vi "状态告警区.vi"(11 "数组":u16[](array[numeric]) format="%04xH") -> (2 "状态告警区 2":T1 {"工作状态" items=["空闲"=0, "水样测试"=1, "标样核查"=2, "零点核查"=3, "跨度核查"=4, "空白测试"=5, "平行样测试"=6, "加标回收"=7, "空白校准"=8, "标样校准"=9, "初始化（清洗）"=10, "单步调试"=254, "简易步骤"=255]; "告警代码" items=["无告警", "缺试剂告警", "缺水样告警", "缺蒸馏水告警", "缺标液告警", "仪表漏液告警", "标定异常告警", "超量程告警", "加热异常", "低试剂预警", "超上限告警", "超下限告警", "仪表内部其他异常", "滴定异常告警", "电极异常告警", "量程切换告警", "参数设置告警", "PH电极电位异常", "电导率电极异常", "浊度光度异常", "溶解氧电极异常", "溶解氧光强异常", "温度异常告警", "PH异常告警", "溶解氧异常告警", "电导率异常告警", "浊度异常告警", "叶绿素异常告警", "藻密度异常告警", "蓝绿藻异常告警", "ORP异常告警", "氨氮异常告警", "清洁刷异常告警", "SD卡异常告警", "蓝牙异常告警", "Wifi异常告警", "流程异常告警"]; "故障代码" items=["无故障", "电机故障", "温度故障", "通讯故障", "滴定故障"]}, 3 "状态告警区":T2 {"工作状态" items=["空闲"=0, "水样测试"=1, "标样核查"=2, "零点核查"=3, "跨度核查"=4, "空白测试"=5, "平行样测试"=6, "加标回收"=7, "空白校准"=8, "标样校准"=9, "初始化（清洗）"=10, "单步调试"=254, "简易步骤"=255]; "告警代码" items=["无告警", "缺试剂告警", "缺水样告警", "缺蒸馏水告警", "缺标液告警", "仪表漏液告警", "标定异常告警", "超量程告警", "加热异常", "低试剂预警", "超上限告警", "超下限告警", "仪表内部其他异常", "滴定异常告警", "电极异常告警", "量程切换告警", "参数设置告警", "PH电极电位异常", "电导率电极异常", "浊度光度异常", "溶解氧电极异常", "溶解氧光强异常", "温度异常告警", "PH异常告警", "溶解氧异常告警", "电导率异常告警", "浊度异常告警", "叶绿素异常告警", "藻密度异常告警", "蓝绿藻异常告警", "ORP异常告警", "氨氮异常告警", "清洁刷异常告警", "SD卡异常告警", "蓝牙异常告警", "Wifi异常告警", "流程异常告警"]; "故障代码" items=["无故障", "电机故障", "温度故障", "通讯故障", "滴定故障"]})   [LabVIEW 2016, in "斯坦道总磷总氮.lvlib"]
panel:
  # "共占用29 WORD"
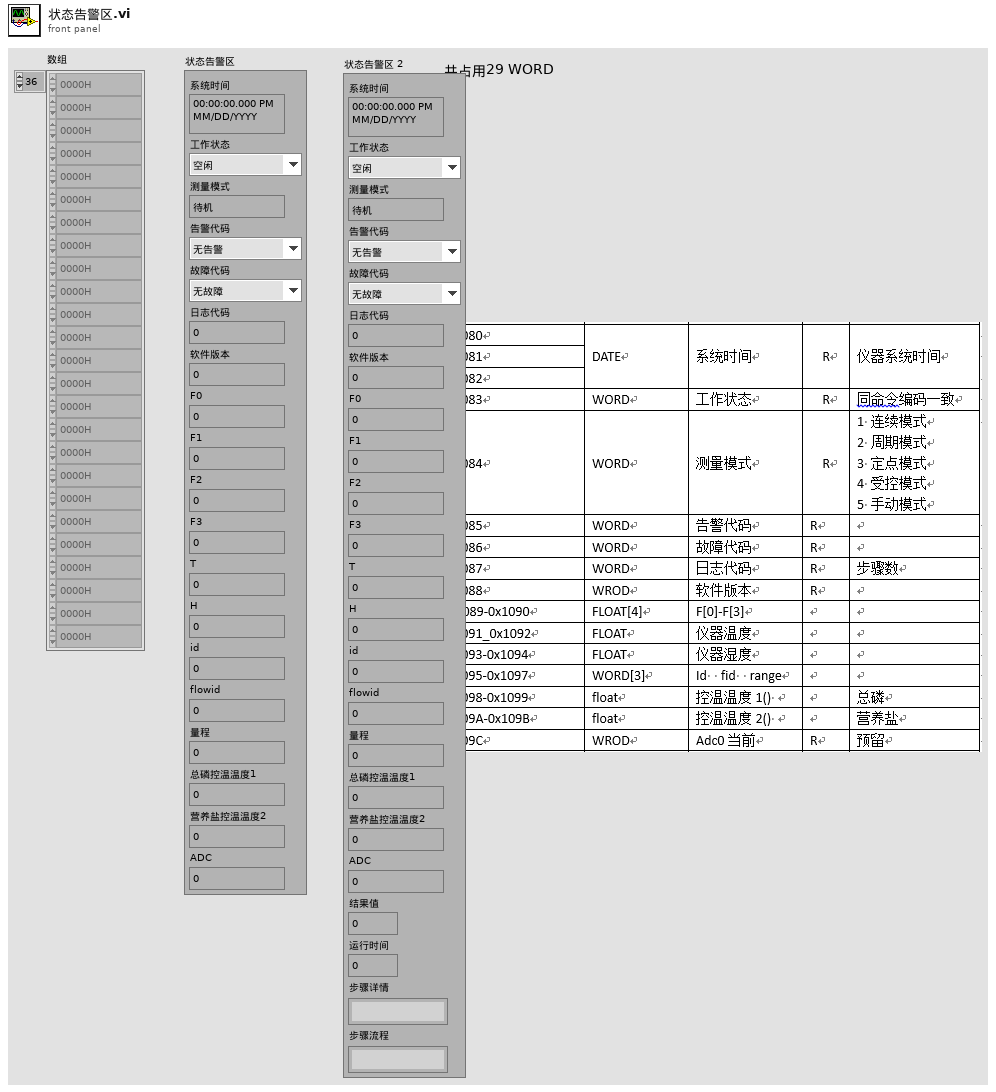
[diagram p1: front panel]
types:
  T1 = cluster{"系统时间":timestamp, "工作状态":u16, "测量模式":enum16{"待机", "连续模式", "周期模式", "定点模式", "受控模式", "手动模式"}, "告警代码":u16, "故障代码":u16, "日志代码":u16, "软件版本":u16, "F0":sgl, "F1":sgl, "F2":sgl, "F3":sgl, "T":sgl, "H":sgl, "id":u16, "flowid":u16, "量程":u16, "总磷控温温度1":sgl, "营养盐控温温度2":sgl, "ADC":sgl, "结果值":sgl, "运行时间":u16, "步骤详情":string, "步骤流程":string}
  T2 = cluster{"系统时间":timestamp, "工作状态":u16, "测量模式":enum16{"待机", "连续模式", "周期模式", "定点模式", "受控模式", "手动模式"}, "告警代码":u16, "故障代码":u16, "日志代码":u16, "软件版本":u16, "F0":sgl, "F1":sgl, "F2":sgl, "F3":sgl, "T":sgl, "H":sgl, "id":u16, "flowid":u16, "量程":u16, "总磷控温温度1":sgl, "营养盐控温温度2":sgl, "ADC":sgl}
  T3 = enum16{"待机", "连续模式", "周期模式", "定点模式", "受控模式", "手动模式"}
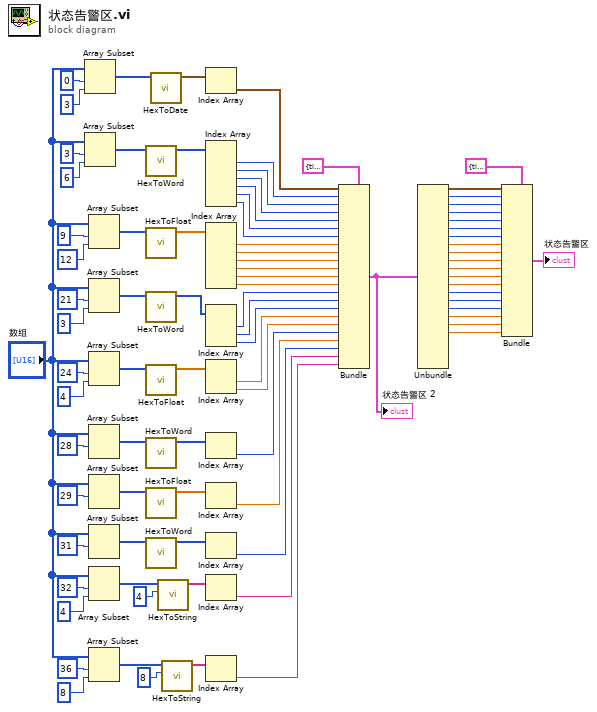
[diagram p0: block diagram]
diagram:
  n1 = Array Subset(array="数组", index=0 ("索引"), length=3 ("长度")) -> (w84:u16[])
  n2 = Array Subset(array="数组", index=3 ("索引"), length=6 ("长度")) -> (w79:u16[])
  n3 = Array Subset(array="数组", index=9 ("索引"), length=12 ("长度")) -> (w69:u16[])
  n4 = Array Subset(array="数组", index=21 ("索引"), length=3 ("索引")) -> (w59:u16[])
  n5 = Array Subset(array="数组", index=24 ("索引"), length=4 ("索引")) -> (w52:u16[])
  n6 = Array Subset(array="数组", index=28 ("索引")) -> (w47:u16[])  [unwired: 1 in]
  n7 = Array Subset(array="数组", index=29 ("索引")) -> (w20:u16[])  [unwired: 1 in]
  n8 = Array Subset(array="数组", index=31 ("索引")) -> (w16:u16[])  [unwired: 1 in]
  n9 = Array Subset(array="数组", index=32 ("索引"), length=4 ("长度")) -> (w12:u16[])
  n10 = Array Subset(array="数组", index=36 ("索引"), length=8 ("长度")) -> (w4:u16[])
  n11 = call "HexToWord.vi"("数组"=w79) -> ("WORD"=w78:u16[])  [unwired: 10 in]
  n12 = call "HexToFloat.vi"("数组"=w69) -> ("FLOAT"=w68:sgl[])  [unwired: 10 in]
  n13 = call "HexToWord.vi"("数组"=w59) -> ("WORD"=w58:u16[])  [unwired: 10 in]
  n14 = call "HexToFloat.vi"("数组"=w52) -> ("FLOAT"=w51:sgl[])  [unwired: 10 in]
  n15 = call "HexToWord.vi"("数组"=w47) -> ("WORD"=w48:u16[])  [unwired: 10 in]
  n16 = call "HexToFloat.vi"("数组"=w20) -> ("FLOAT"=w19:sgl[])  [unwired: 10 in]
  n17 = call "HexToWord.vi"("数组"=w16) -> ("WORD"=w15:u16[])  [unwired: 10 in]
  n18 = call "HexToDate.vi"("数组"=w84) -> ("DATE"=w81:timestamp[])  [unwired: 10 in]
  n19 = call "HexToString.vi"("字符个数"=4, "数组"=w12) -> ("STRING"=w10:string[])  [unwired: 9 in]
  n20 = call "HexToString.vi"("字符个数"=8, "数组"=w4) -> ("STRING"=w6:string[])  [unwired: 9 in]
  n21 = Index Array(array=w81) -> (element=w80:timestamp)  [unwired: 1 in]
  n22 = Index Array(array=w78) -> (element #1=w77:u16, element #2=w76:u16, element #3=w75:u16, element #4=w74:u16, element #5=w73:u16, element #6=w72:u16)  [unwired: 6 in]
  n23 = Index Array(array=w68) -> (element #1=w67:sgl, element #2=w66:sgl, element #3=w65:sgl, element #4=w64:sgl, element #5=w63:sgl, element #6=w62:sgl)  [unwired: 6 in]
  n24 = Index Array(array=w58) -> (element #1=w57:u16, element #2=w56:u16, element #3=w55:u16)  [unwired: 3 in]
  n25 = Index Array(array=w51) -> (element #1=w50:sgl, element #2=w49:sgl)  [unwired: 2 in]
  n26 = Index Array(array=w48) -> (element=w45:u16)  [unwired: 1 in]
  n27 = Index Array(array=w19) -> (element=w18:sgl)  [unwired: 1 in]
  n28 = Index Array(array=w15) -> (element=w14:u16)  [unwired: 1 in]
  n29 = Index Array(array=w10) -> (element=w9:string)  [unwired: 1 in]
  n30 = Index Array(array=w6) -> (element=w1:string)  [unwired: 1 in]
  n31 = Bundle(cluster=T1 {"系统时间"=timestamp(0 s since 1904-01-01), "工作状态"=0, "测量模式"=enum."待机", "告警代码"=0, "故障代码"=0, "日志代码"=0, "软件版本"=0, "F0"=0.0, "F1"=0.0, "F2"=0.0, "F3"=0.0, "T"=0.0, "H"=0.0, "id"=0, "flowid"=0, "量程"=0, "总磷控温温度1"=0.0, "营养盐控温温度2"=0.0, "ADC"=0.0, "结果值"=0.0, "运行时间"=0, "步骤详情"="", "步骤流程"=""} ("状态告警区 2"), "系统时间"=w80, "工作状态"=w77, "测量模式"=w76, "告警代码"=w75, "故障代码"=w74, "日志代码"=w73, "软件版本"=w72, "F0"=w67, "F1"=w66, "F2"=w65, "F3"=w64, "T"=w63, "H"=w62, "id"=w57, "flowid"=w56, "量程"=w55, "总磷控温温度1"=w50, "营养盐控温温度2"=w49, "ADC"=w45, "结果值"=w18, "运行时间"=w14, "步骤详情"=w9, "步骤流程"=w1) -> (w43:T1)
  "状态告警区 2" <- w43
  n32 = Unbundle(w43) -> ("系统时间"=w41:timestamp, "工作状态"=w40:u16, "测量模式"=w39:T3, "告警代码"=w38:u16, "故障代码"=w37:u16, "日志代码"=w36:u16, "软件版本"=w35:u16, "F0"=w34:sgl, "F1"=w33:sgl, "F2"=w32:sgl, "F3"=w31:sgl, "T"=w30:sgl, "H"=w29:sgl, "id"=w28:u16, "flowid"=w27:u16, "量程"=w26:u16, "总磷控温温度1"=w25:sgl, "营养盐控温温度2"=w24:sgl, "ADC"=w23:sgl)  [unwired: 4 out]
  n33 = Bundle(cluster=T2 {"系统时间"=timestamp(0 s since 1904-01-01), "工作状态"=0, "测量模式"=enum."待机", "告警代码"=0, "故障代码"=0, "日志代码"=0, "软件版本"=0, "F0"=0.0, "F1"=0.0, "F2"=0.0, "F3"=0.0, "T"=0.0, "H"=0.0, "id"=0, "flowid"=0, "量程"=0, "总磷控温温度1"=0.0, "营养盐控温温度2"=0.0, "ADC"=0.0} ("状态告警区"), "系统时间"=w41, "工作状态"=w40, "测量模式"=w39, "告警代码"=w38, "故障代码"=w37, "日志代码"=w36, "软件版本"=w35, "F0"=w34, "F1"=w33, "F2"=w32, "F3"=w31, "T"=w30, "H"=w29, "id"=w28, "flowid"=w27, "量程"=w26, "总磷控温温度1"=w25, "营养盐控温温度2"=w24, "ADC"=w23) -> (→"状态告警区":T2)
